vi "DSF.Engine.Plugin.Shutdown (old).vi"(8 "error in (no error)":errorcluster, 11 "Plugin in":refnum<class "DSF.Engine.Plugin.lvclass">) -> (0 "error out":errorcluster, 3 "Plugin out":refnum<class "DSF.Engine.Plugin.lvclass">)   [LabVIEW 2017, in "DSF.Engine.lvlib" / "DSF.Engine.Plugin.lvclass"]
uses:
  DSF.Engine.Plugin.lvclass
  DSF.Engine.Plugin.lvclass/DSF.Engine.Plugin.ctl
  Transceiver/DSF.Engine.Transceiver.lvclass
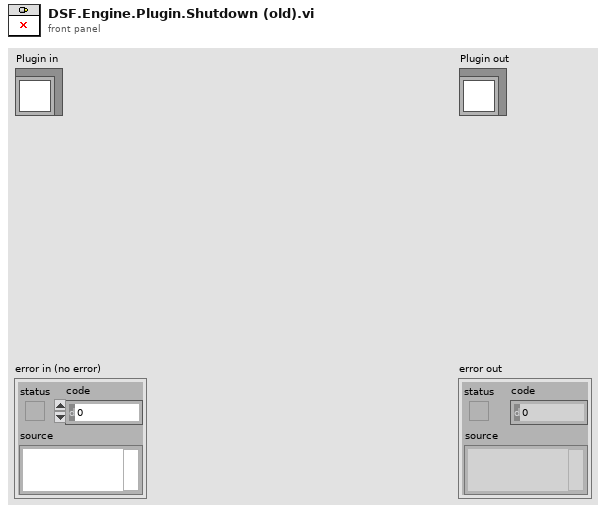
[diagram p1: front panel]
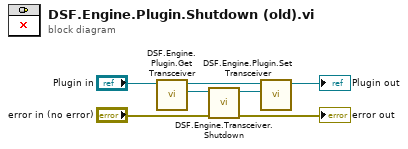
[diagram p0: block diagram]
diagram:
  n1 = call "DSF.Engine.Plugin.Get Transceiver.vi"("Plugin in"="Plugin in") -> ("Transceiver"=w7:refnum<class "DSF.Engine.Transceiver.lvclass">, "Plugin out"=w5:refnum<class "DSF.Engine.Plugin.lvclass">)  [unwired: 9 in]
  n2 = call-dynamic "DSF.Engine.Transceiver.Shutdown.vi"("error in (no error)"="error in (no error)", "Transceiver in"=w7) -> ("error out"=→"error out":errorcluster, "Transceiver out"=w6:refnum<class "DSF.Engine.Transceiver.lvclass">)  [unwired: 8 in]
  n3 = call "DSF.Engine.Plugin.Set Transceiver.vi"("Transceiver"=w6, "Plugin in"=w5) -> ("Plugin out"=→"Plugin out":refnum<class "DSF.Engine.Plugin.lvclass">)  [unwired: 9 in]
